vi "Pop_up.vi"() -> ()   [LabVIEW 2020]
doc: "This Vi is used as a popup vi which is started with an invoke node from the main vi"
panel:
  in  "Boolean":bool
  # "Click this button to stop the execution of the VI"
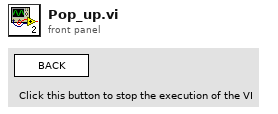
[diagram p1: front panel]
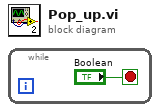
[diagram p0: block diagram]
diagram:
  n1 = while {
    stop <- "Boolean" stop-if-true
  }
